vi "crd_fitTau.vi"(9 "y Data (volts)":dbl[][](array[numeric]), 10 "Sample Internal":sgl) -> (2 "tau (us)":dbl, 3 "Decay":cluster{sgl[], "Best Exponential Fit":dbl[]}[](graph))   [LabVIEW 2011]
uses:
  <vilib>/Analysis/NI_AALPro.lvlib
  <vilib>/Analysis/NI_AALBase.lvlib
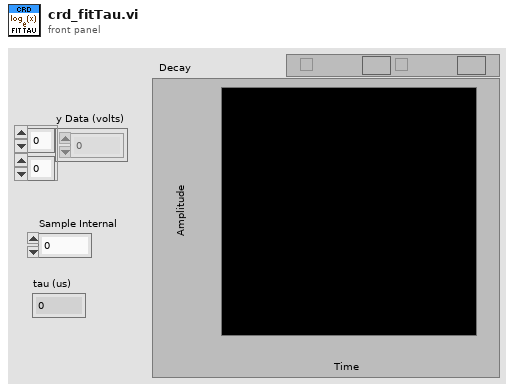
[diagram p1: front panel]
types:
  T1 = cluster{"amp min":dbl, "amp max":dbl, "damping min":dbl, "damping max":dbl, "offset min":dbl, "offset max":dbl}
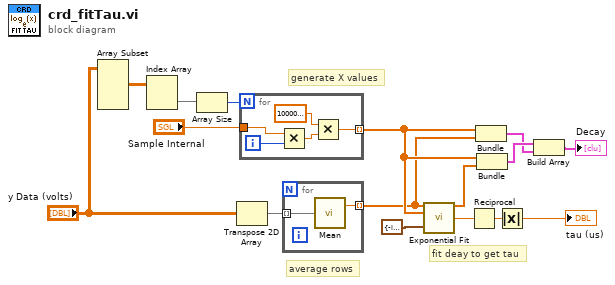
[diagram p0: block diagram]
diagram:
  # "generate X values"
  # "fit deay to get tau"
  # "average rows"
  n1 = Array Subset(array="y Data (volts)") -> (w7:dbl[][])  [unwired: 4 in]
  n2 = Index Array(array=w7) -> (element=w6:dbl[])  [unwired: 2 in]
  n3 = Array Size(array=w6) -> (size(s)=w16:i32)
  n4 = Transpose 2D Array(2D array="y Data (volts)") -> (transposed array=w12:dbl[][])
  n5 = for {
    N: w16 -> [_]
    tunnel: [w19] -> w11 mode=indexing
    tunnel: "Sample Internal" -> [w17]
    i -> [w21]
    n6 = Multiply(x=w17, y=w21) -> (x*y=w20:sgl)
    n7 = Multiply(x=sgl 1000000.0, y=w20) -> (x*y=w19:sgl)
  }
  n8 = for {
    tunnel: w12 -> [w23] mode=indexing
    tunnel: [w22] -> w2 mode=indexing
    n9 = call <vilib>:"Mean.vi"("X"=w23) -> ("mean"=w22:dbl)  [unwired: 1 out]
  }
  n10 = call <vilib>:"Exponential Fit.vi"("Y"=w2, "X"=w11, "parameter bounds"=T1 {"amp min"=-inf, "amp max"=inf, "damping min"=-inf, "damping max"=inf, "offset min"=0.0, "offset max"=10.0}) -> ("Best Exponential Fit"=w10:dbl[], "damping"=w13:dbl)  [unwired: 7 in, 4 out]
  n11 = Reciprocal(x=w13) -> (1/x=w14:dbl)
  n12 = Bundle(w11, w2) -> (w3:cluster{sgl[], dbl[]})  [unwired: 1 in]
  n13 = Bundle(w11, "Best Exponential Fit"=w10) -> (w4:cluster{sgl[], "Best Exponential Fit":dbl[]})  [unwired: 1 in]
  n14 = Absolute Value(x=w14) -> (abs(x)=→"tau (us)":dbl)
  n15 = Build Array(w4, w3) -> (→"Decay":cluster{sgl[], "Best Exponential Fit":dbl[]}[])
